vi "CRYUpdate Receiver Index.vi"(8 "Chn Idx":i32, 10 "Receiver_Index":i32) -> ()   [LabVIEW 2013]
uses:
  CRYMisc vis settings global.vi
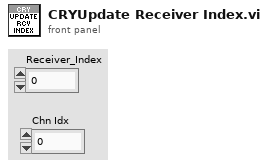
[diagram p1: front panel]
types:
  T1 = cluster{"Rcv Idx":i32, "Chn Idx":i32, "Data":i32[], "bufCount":i32}[]
  T2 = cluster{"Rcv Idx":i32, "Chn Idx":i32, "Data":i32[], "bufCount":i32}
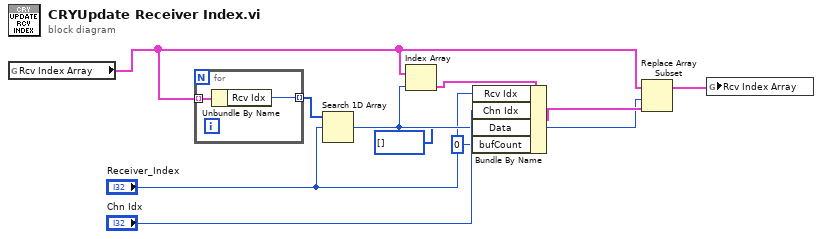
[diagram p0: block diagram]
diagram:
  n1 = global read "CRYMisc vis settings global.vi" "Rcv Index Array"() -> (w5:T1)
  n2 = for {
    tunnel: w5 -> [w12] mode=indexing
    tunnel: [w11] -> w10 mode=indexing
    n3 = Unbundle By Name(w12) -> ("Rcv Idx"=w11:i32)
  }
  n4 = Search 1D Array(1D array=w10, element="Receiver_Index") -> (index of element=w6:i32)  [unwired: 1 in]
  n5 = Index Array(array=w5, index=w6) -> (element=w9:T2)
  n6 = Bundle By Name(cluster=w9, "Rcv Idx"="Receiver_Index", "Chn Idx"="Chn Idx", "Data"=i32[] [], "bufCount"=0) -> (w7:T2)
  n7 = Replace Array Subset(array=w5, new element=w7, index=w6) -> (w4:T1)
  n8 = global write "CRYMisc vis settings global.vi" "Rcv Index Array"(w4) -> ()
